vi "publisher state machine.vi"(8 "results reporter":refnum<class "results reporter.lvclass">, 9 "execution system":T1=enum."standard", 10 "thread pool":refnum<class "thread pool.lvclass">, 11 "starburst in":refnum<class "publisher.lvclass">) -> ()   [LabVIEW 2015, in "publisher.lvclass"]
uses:
  publisher.lvclass
  taskpool/dispatcher/thread pool.lvclass
  taskpool/dispatcher/execution system.ctl
  taskpool/results reporter/results reporter.lvclass
  communicator queue/identifying queue.lvclass
  registered subscriptions.ctl
  communicator/communicator.lvclass/communicator.ctl
  communicator queue/identifying queue.lvclass/identifying queue.ctl
  message/communicator message.lvclass/communicator message.ctl
  communicator queue/enqueue variety.ctl
  message/set sender.vi
  message/communicator message.lvclass
  connection/connection maintainer.lvclass
  communicator/communicator.lvclass
  manager/queue manager.lvclass
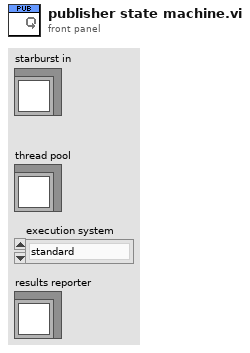
[diagram p1: front panel]
types:
  T1 = typedef "thread pool.lvclass/execution system.ctl" = enum32{"user interface", "standard", "instrument i/o", "data acquisition", "other 1", "other 2"}
  T2 = typedef "publisher.lvclass/registered subscriptions.ctl" = cluster{"patterns":string[], "connections":cluster{"connections":refnum<class "identifying queue.lvclass">[]}[]}
  T3 = typedef "identifying queue.lvclass/enqueue variety.ctl" = enum16{"normal", "lossy", "priority"}
  T4 = cluster{"connections":refnum<class "identifying queue.lvclass">[]}[]
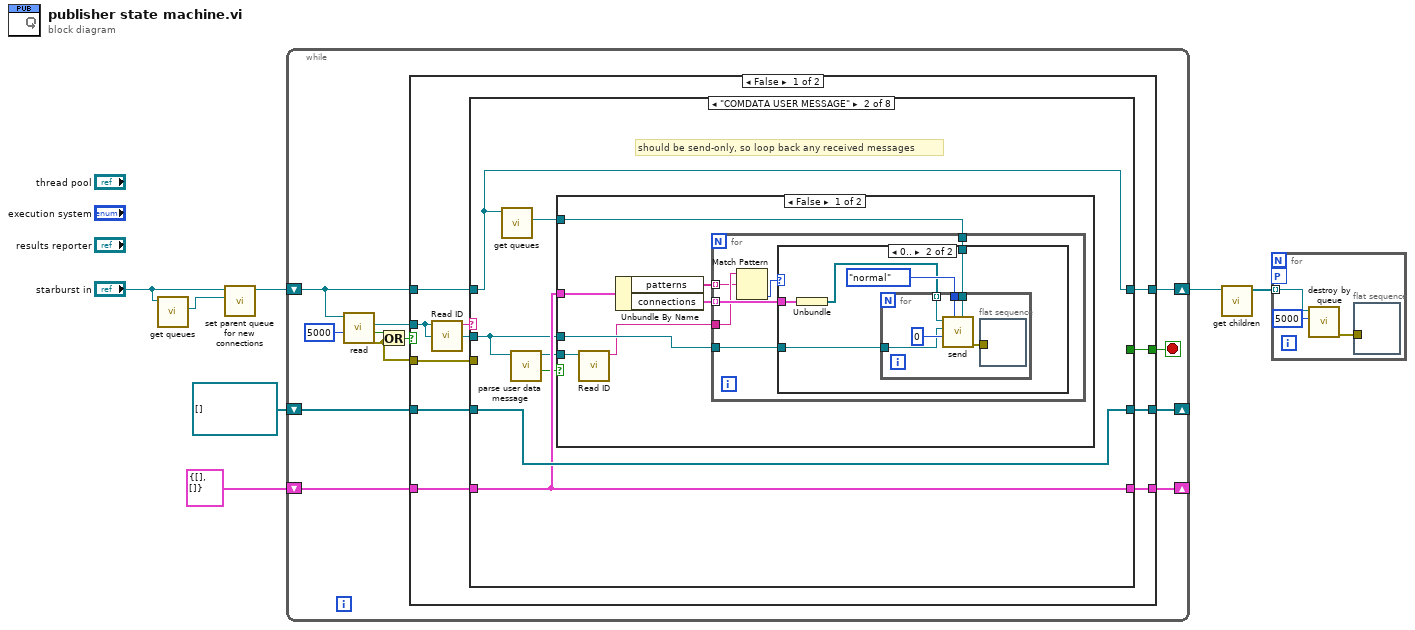
[diagram p0: block diagram]
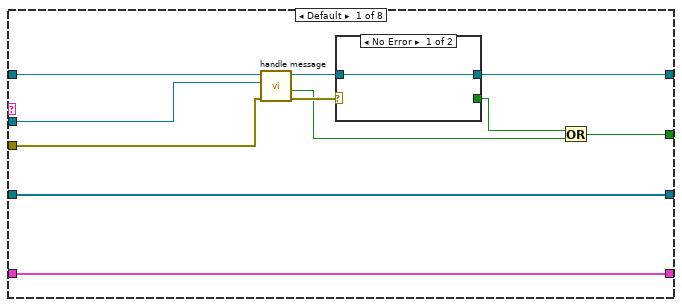
[diagram p2: hidden frame]
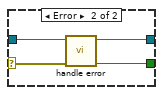
[diagram p3: hidden frame]
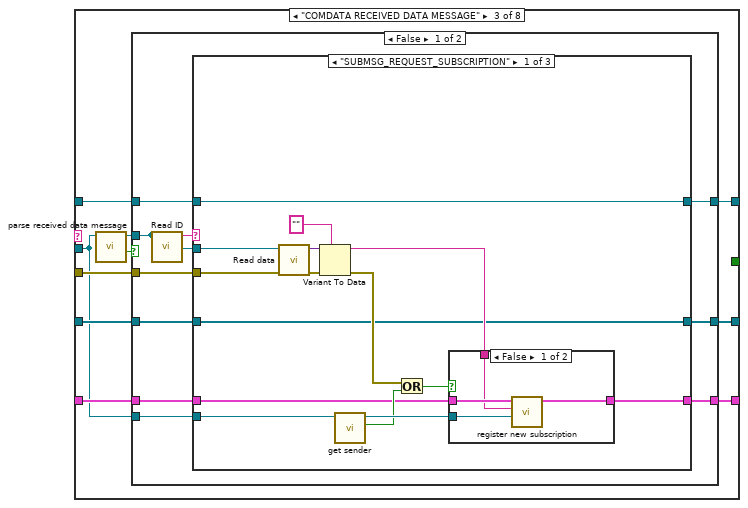
[diagram p6: hidden frame]
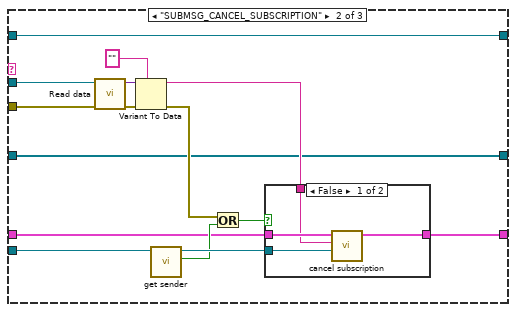
[diagram p8: hidden frame]
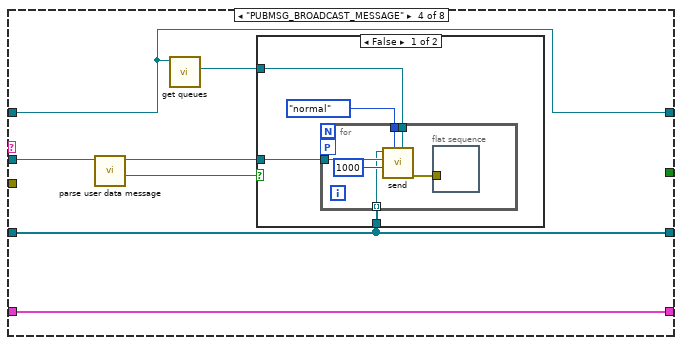
[diagram p12: hidden frame]
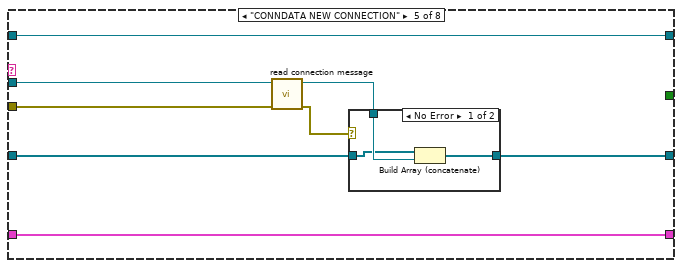
[diagram p14: hidden frame]
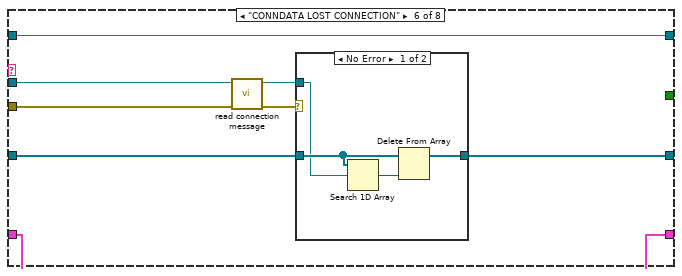
[diagram p16: hidden frame]
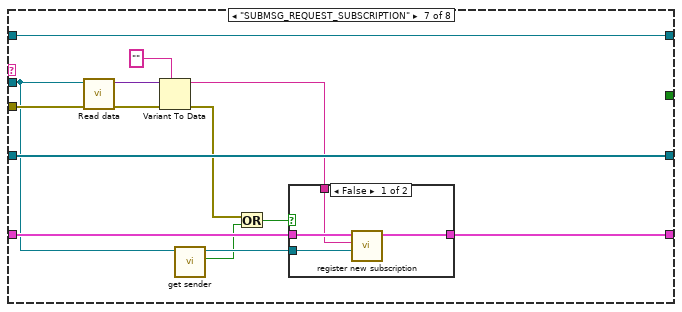
[diagram p18: hidden frame]
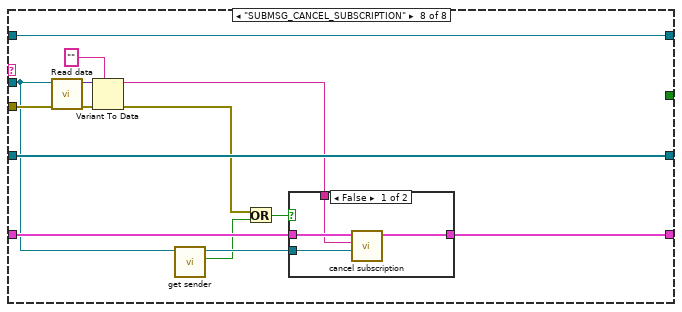
[diagram p20: hidden frame]
diagram:
  n1 = call "get queues.vi"("communicator in"="starburst in") -> ("to this"=w1:refnum<class "identifying queue.lvclass">)  [unwired: 9 in, 1 out]
  n2 = call "set parent queue for new connections.vi"("conn parent queue"=w1, "queue manager in"="starburst in") -> ("queue manager out"=w3:refnum<class "publisher.lvclass">)  [unwired: 9 in]
  n3 = while {
    shift-right: [w17] -> _
    shift-left: refnum<class "identifying queue.lvclass">[] [] -> [w16]
    shift-right: [w15] -> _
    shift-left: T2 {"patterns"=[], "connections"=[]} ("registered subscriptions out") -> [w14]
    shift-right: [w10] -> w5
    shift-left: w3 -> [w9]
    stop <- w18 stop-if-true
    n4 = call "read.vi"("timeout in ms (-1)"=5000, "communicator in"=w9) -> ("error out"=w11:errorcluster, "timed out?"=w13:bool, "message"=w12:refnum<class "communicator message.lvclass">)  [unwired: 7 in]
    n5 = Or(x=w13, y=w11) -> (x .or. y?=w19:bool)
    n6 = case shown="False" w19 {
      tunnel: w11 -> [w27 w227]
      tunnel: [w20 w220] -> w18
      tunnel: w12 -> [w28 _]
      tunnel: [w26 w226] -> w17
      tunnel: w16 -> [w25 w226]
      tunnel: [w24 w225] -> w15
      tunnel: w14 -> [w23 w225]
      tunnel: w9 -> [w22 w221]
      tunnel: [w21 w221] -> w10
      frame False {
        n7 = call "Read ID.vi"("communicator message in"=w28) -> ("ID"=w29:string)  [unwired: 10 in]
        n8 = case shown="\"COMDATA USER MESSAGE\"" w29 {
          tunnel: w28 -> [w34 w48 w77 w145 w158 w176 w187 w206]
          tunnel: w27 -> [w33 _ w84 _ w165 w177 w193 w211]
          tunnel: [w39 w52 w81 w147 w163 w174 w195 w213] -> w26
          tunnel: w25 -> [w39 w52 w80 w147 w162 w173 w195 w213]
          tunnel: [w40 w51 w78 w146 w160 w171 w192 w210] -> w24
          tunnel: w23 -> [w40 w51 w79 w146 w160 w171 w191 w209]
          tunnel: w22 -> [w38 w50 w83 w142 w159 w170 w185 w204]
          tunnel: [w37 w50 w82 w142 w159 w170 w185 w204] -> w21
          tunnel: [w32 _ _ _ _ _ _ _] -> w20
          frame Default {
            n9 = call-dynamic "handle message.vi"("error in"=w33, "message"=w34, "queue manager in"=w38) -> ("error out"=w35:errorcluster, "stop"=w31:bool, "queue manager out"=w36:refnum<class "publisher.lvclass">)  [unwired: 6 in]
            n10 = case shown="No Error" w35 {
              selector: w35 -> [_ w43]
              tunnel: [w41 w44] -> w37
              tunnel: w36 -> [w41 w45]
              tunnel: [_ w42] -> w30
              frame No Error {
              }
              frame Error {
                n11 = call-dynamic "handle error.vi"("error in"=w43, "communicator in"=w45) -> ("unrecoverable?"=w42:bool, "communicator out"=w44:refnum<class "publisher.lvclass">)  [unwired: 8 in]
              }
            }
            n12 = Or(x=w30, y=w31) -> (x .or. y?=w32:bool)
          }
          frame "COMDATA USER MESSAGE" {
            # "should be send-only, so loop back any received messages"
            n13 = call "get queues.vi"("communicator in"=w50) -> ("to this"=w49:refnum<class "identifying queue.lvclass">)  [unwired: 9 in, 1 out]
            n14 = call "parse user data message.vi"("message"=w48) -> ("invalid?"=w47:bool, "data"=w46:refnum<class "communicator message.lvclass">)  [unwired: 9 in]
            n15 = case shown="False" w47 {
              tunnel: w51 -> [w59 _]
              tunnel: w49 -> [w58 _]
              tunnel: w48 -> [w55 _]
              tunnel: w46 -> [w54 _]
              frame False {
                n16 = call "Read ID.vi"("communicator message in"=w54) -> ("ID"=w53:string)  [unwired: 10 in]
                n17 = Unbundle By Name(w59) -> ("patterns"=w57:string[], "connections"=w56:T4)
                n18 = for {
                  tunnel: w53 -> [w62]
                  tunnel: w57 -> [w61] mode=indexing
                  tunnel: w56 -> [w64] mode=indexing
                  tunnel: w55 -> [w63]
                  tunnel: w58 -> [w60]
                  n19 = Match Pattern(string=w62, regular expression=w61) -> (offset past match=w65:i32)  [unwired: 1 in, 3 out]
                  n20 = case shown="0.." w65 {
                    tunnel: w64 -> [_ w70]
                    tunnel: w63 -> [_ w67]
                    tunnel: w60 -> [_ w66]
                    frame ..-1 {
                    }
                    frame 0.. {
                      n21 = Unbundle(w70) -> ("connections"=w68:refnum<class "identifying queue.lvclass">[])
                      n22 = for {
                        tunnel: enqueue_variety."normal" ("enqueue setting") -> [w76]
                        tunnel: w68 -> [w74] mode=indexing
                        tunnel: w67 -> [w73]
                        tunnel: w66 -> [w71]
                        n23 = call "send.vi"("sender"=w71, "enqueue command"=w76, "timeout in ms (-1)"=0, "message"=w73, "message connection in"=w74) -> ("error out"=w72:errorcluster)  [unwired: 5 in, 1 out]
                        n24 = flat-sequence {
                          tunnel: w72 -> [_]
                          frame #0 {
                          }
                        }
                      }
                    }
                  }
                }
              }
              frame True {
              }
            }
          }
          frame "COMDATA RECEIVED DATA MESSAGE" {
            n25 = call "parse received data message.vi"("message"=w77) -> ("invalid?"=w86:bool, "data"=w85:refnum<class "communicator message.lvclass">)  [unwired: 9 in]
            n26 = case shown="False" w86 {
              tunnel: w85 -> [w89 _]
              tunnel: w84 -> [w88 _]
              tunnel: w83 -> [w94 w140]
              tunnel: [w95 w140] -> w82
              tunnel: [w92 w139] -> w81
              tunnel: w80 -> [w93 w139]
              tunnel: w79 -> [w90 w138]
              tunnel: [w91 w138] -> w78
              tunnel: w77 -> [w87 _]
              frame False {
                n27 = call "Read ID.vi"("communicator message in"=w89) -> ("ID"=w96:string)  [unwired: 10 in]
                n28 = case shown="\"SUBMSG_REQUEST_SUBSCRIPTION\"" w96 {
                  tunnel: [w102 w121 w137] -> w95
                  tunnel: w94 -> [w102 w121 w137]
                  tunnel: w93 -> [w103 w122 w136]
                  tunnel: [w103 w122 w136] -> w92
                  tunnel: [w99 w118 w135] -> w91
                  tunnel: w90 -> [w100 w119 w135]
                  tunnel: w89 -> [w98 w117 _]
                  tunnel: w88 -> [w101 w120 _]
                  tunnel: w87 -> [w97 w116 _]
                  frame "SUBMSG_REQUEST_SUBSCRIPTION" {
                    n29 = call "Read data.vi"("communicator message in"=w98) -> ("data"=w110:variant)  [unwired: 10 in]
                    n30 = Variant To Data(error in=w101, type="", Variant=w110) -> (data=w107:string, error out=w109:errorcluster)
                    n31 = call "get sender.vi"("message in"=w97) -> ("invalid?"=w104:bool, "sender"=w106:refnum<class "identifying queue.lvclass">)  [unwired: 9 in]
                    n32 = Or(x=w109, y=w104) -> (x .or. y?=w105:bool)
                    n33 = case shown="False" w105 {
                      tunnel: [w114 w115] -> w99
                      tunnel: w100 -> [w113 w115]
                      tunnel: w107 -> [w112 _]
                      tunnel: w106 -> [w111 _]
                      frame False {
                        n34 = call "register new subscription.vi"("queue"=w111, "pattern"=w112, "registered subscriptions in"=w113) -> ("registered subscriptions out"=w114:T2)  [unwired: 8 in]
                      }
                      frame True {
                      }
                    }
                  }
                  frame "SUBMSG_CANCEL_SUBSCRIPTION" {
                    n35 = call "Read data.vi"("communicator message in"=w117) -> ("data"=w129:variant)  [unwired: 10 in]
                    n36 = Variant To Data(error in=w120, type="", Variant=w129) -> (data=w126:string, error out=w128:errorcluster)
                    n37 = call "get sender.vi"("message in"=w116) -> ("invalid?"=w123:bool, "sender"=w125:refnum<class "identifying queue.lvclass">)  [unwired: 9 in]
                    n38 = Or(x=w128, y=w123) -> (x .or. y?=w124:bool)
                    n39 = case shown="False" w124 {
                      tunnel: [w133 w134] -> w118
                      tunnel: w119 -> [w132 w134]
                      tunnel: w126 -> [w131 _]
                      tunnel: w125 -> [w130 _]
                      frame False {
                        n40 = call "cancel subscription.vi"("queue"=w130, "pattern"=w131, "registered subscriptions in"=w132) -> ("registered subscriptions out"=w133:T2)  [unwired: 8 in]
                      }
                      frame True {
                      }
                    }
                  }
                  frame Default {
                  }
                }
              }
              frame True {
              }
            }
          }
          frame "PUBMSG_BROADCAST_MESSAGE" {
            n41 = call "parse user data message.vi"("message"=w145) -> ("invalid?"=w143:bool, "data"=w144:refnum<class "communicator message.lvclass">)  [unwired: 9 in]
            n42 = call "get queues.vi"("communicator in"=w142) -> ("to this"=w141:refnum<class "identifying queue.lvclass">)  [unwired: 9 in, 1 out]
            n43 = case shown="False" w143 {
              tunnel: w147 -> [w151 _]
              tunnel: w144 -> [w149 _]
              tunnel: w141 -> [w148 _]
              frame False {
                n44 = for {
                  workers-P: _ -> [_]
                  tunnel: w149 -> [w157]
                  tunnel: enqueue_variety."normal" ("enqueue setting") -> [w156]
                  tunnel: w151 -> [w153] mode=indexing
                  tunnel: w148 -> [w152]
                  n45 = call "send.vi"("sender"=w152, "enqueue command"=w156, "timeout in ms (-1)"=1000, "message"=w157, "message connection in"=w153) -> ("error out"=w154:errorcluster)  [unwired: 5 in, 1 out]
                  n46 = flat-sequence {
                    tunnel: w154 -> [_]
                    frame #0 {
                    }
                  }
                }
              }
              frame True {
              }
            }
          }
          frame "CONNDATA NEW CONNECTION" {
            n47 = call "read connection message.vi"("error in"=w165, "communicator message in"=w158) -> ("error out"=w161:errorcluster, "queue"=w164:refnum<class "identifying queue.lvclass">)  [unwired: 8 in]
            n48 = case shown="No Error" w161 {
              tunnel: w164 -> [w168 _]
              tunnel: [w167 w169] -> w163
              tunnel: w162 -> [w166 w169]
              frame No Error {
                n49 = Build Array (concatenate)(w166, w168) -> (w167:refnum<class "identifying queue.lvclass">[])
              }
              frame Error {
              }
            }
          }
          frame "CONNDATA LOST CONNECTION" {
            n50 = call "read connection message.vi"("error in"=w177, "communicator message in"=w176) -> ("error out"=w175:errorcluster, "queue"=w172:refnum<class "identifying queue.lvclass">)  [unwired: 8 in]
            n51 = case shown="No Error" w175 {
              tunnel: [w179 w182] -> w174
              tunnel: w173 -> [w180 w182]
              tunnel: w172 -> [w178 _]
              frame No Error {
                n52 = Search 1D Array(1D array=w180, element=w178) -> (index of element=w181:i32)  [unwired: 1 in]
                n53 = Delete From Array(array=w180, index=w181) -> (array with subset deleted=w179:refnum<class "identifying queue.lvclass">[])  [unwired: 1 in, 1 out]
              }
              frame Error {
              }
            }
          }
          frame "SUBMSG_REQUEST_SUBSCRIPTION" {
            n54 = call "Read data.vi"("communicator message in"=w187) -> ("data"=w194:variant)  [unwired: 10 in]
            n55 = Variant To Data(error in=w193, type="", Variant=w194) -> (data=w188:string, error out=w190:errorcluster)
            n56 = call "get sender.vi"("message in"=w187) -> ("invalid?"=w183:bool, "sender"=w186:refnum<class "identifying queue.lvclass">)  [unwired: 9 in]
            n57 = Or(x=w190, y=w183) -> (x .or. y?=w184:bool)
            n58 = case shown="False" w184 {
              tunnel: [w199 w200] -> w192
              tunnel: w191 -> [w198 w200]
              tunnel: w188 -> [w197 _]
              tunnel: w186 -> [w196 _]
              frame False {
                n59 = call "register new subscription.vi"("queue"=w196, "pattern"=w197, "registered subscriptions in"=w198) -> ("registered subscriptions out"=w199:T2)  [unwired: 8 in]
              }
              frame True {
              }
            }
          }
          frame "SUBMSG_CANCEL_SUBSCRIPTION" {
            n60 = call "Read data.vi"("communicator message in"=w206) -> ("data"=w212:variant)  [unwired: 10 in]
            n61 = Variant To Data(error in=w211, type="", Variant=w212) -> (data=w207:string, error out=w201:errorcluster)
            n62 = call "get sender.vi"("message in"=w206) -> ("invalid?"=w202:bool, "sender"=w205:refnum<class "identifying queue.lvclass">)  [unwired: 9 in]
            n63 = Or(x=w201, y=w202) -> (x .or. y?=w203:bool)
            n64 = case shown="False" w203 {
              tunnel: [w217 w218] -> w210
              tunnel: w209 -> [w216 w218]
              tunnel: w207 -> [w215 _]
              tunnel: w205 -> [w214 _]
              frame False {
                n65 = call "cancel subscription.vi"("queue"=w214, "pattern"=w215, "registered subscriptions in"=w216) -> ("registered subscriptions out"=w217:T2)  [unwired: 8 in]
              }
              frame True {
              }
            }
          }
        }
      }
      frame True {
        n66 = Unbundle By Name(w227) -> ("status"=w224:bool)
        n67 = call "get queues.vi"("communicator in"=w221) -> ("to parent"=w223:refnum<class "identifying queue.lvclass">)  [unwired: 9 in, 1 out]
        n68 = call "is valid.vi"("identifying queue in"=w223) -> ("valid?"=w222:bool)  [unwired: 9 in, 1 out]
        n69 = Not(x=w222) -> (.not. x?=w219:bool)
        n70 = Or(x=w219, y=w224) -> (x .or. y?=w220:bool)
      }
    }
  }
  n71 = call "get children.vi"("communicator in"=w5) -> ("children"=w4:refnum<class "identifying queue.lvclass">[])  [unwired: 10 in]
  n72 = for {
    workers-P: _ -> [_]
    tunnel: w4 -> [w228] mode=indexing
    n73 = call "destroy by queue.vi"("timeout in ms (-1)"=5000, "queue"=w228) -> ("error out"=w229:errorcluster)  [unwired: 8 in, 1 out]
    n74 = flat-sequence {
      tunnel: w229 -> [_]
      frame #0 {
      }
    }
  }
